vi "Global_All_Data.vi"() -> ()   [LabVIEW 2019]
uses:
  TypeDef/Cluster MISURE.ctl
  TypeDef/MISURE NM.ctl
  TypeDef/Cluster misure ALL.ctl
  TypeDef/Cluster NI.ctl
  cDAQ_PLC Folder/controls/StatoAO_cdaq.ctl
  cDAQ_PLC Folder/controls/statoDO_Cdaq.ctl
  TypeDef/MISURE WT.ctl
  TypeDef/ClusterRes.ctl
  TypeDef/INTERFACCIA.ctl
  TypeDef/Lista AO sistema.ctl
  TypeDef/DOinterfaccia.ctl
  cDAQ_PLC Folder/ST1200_LIST_IO/STATO PLC 1.ctl
  cDAQ_PLC Folder/ST1200_LIST_IO/Uscite PLC 1.ctl
  cDAQ_PLC Folder/controls/statoAO_plc_1.ctl
  cDAQ_PLC Folder/ST1200_LIST_IO/StatoDO_PLC_1.ctl
  SINUS PENTA SANTERNO/controls/Parametri inverter letti.ctl
  cDAQ_PLC Folder/ST1200_LIST_IO/STATO PLC 2.ctl
  cDAQ_PLC Folder/ST1200_LIST_IO/Uscite PLC 2.ctl
  cDAQ_PLC Folder/controls/statoAO_plc_2.ctl
  cDAQ_PLC Folder/ST1200_LIST_IO/StatoDO_PLC_2.ctl
  cDAQ_PLC Folder/ST1200_LIST_IO/STATO PLC 3.ctl
  cDAQ_PLC Folder/ST1200_LIST_IO/Uscite PLC 3.ctl
  cDAQ_PLC Folder/controls/statoAO_plc_3.ctl
  cDAQ_PLC Folder/ST1200_LIST_IO/StatoDO_PLC_3.ctl
  DCREG/Parametri DCREG letti.ctl
panel:
  out "All Data":T1={"MISURE NM"={"Banco"="", "Anno"="", "Numero"="", "Ntabella"="", "Misura"="", "Tipo Prova"="", "ProgressivoAcq"="", "Descrizione"="", "Data_ora"="", "t. acq [h:m:s]"="", "t. acq [min]"="", "t. acq [s]"="", "n [rpm]"="", "f [Hz]"="", "U1[V]"="", "U2 [V]"="", "U3 [V]"="", "U123_media [V]"="", "I1[A]"="", "I2[A]"="", "I3[A]"="", "I123_media [A]*I"="", "I_123_sbil [%]"="", "Ulin[V]"="", "Uc [V]"="", "Uaux [V]"="", "Ilin[A]*I"="", "Imar[A]"="", "Iaux[A]"="", "Uarm[V]"="", "Uecc[V]"="", "Iarm[A]*I"="", "Iecc[A]"="", "pf"="", "P1 [W]"="", "P1 [kW]"="", "Q [VAR]"="", "Q [kVAR]"="", "S [VA]"="", "S [kVA]"="", "P1arm[W]"="", "P1ecc[W]"="", "Parm[kW]"="", "P1ecc[kW]"="", "Cond[uF]"="", "P1_linea_6fili[W]"="", "P1_linea_6fili[kW]"="", "eta_gr_6fili [%]"="", "eta_inverter_6fili [%]"="", "pf_linea_6fili"="", "U4 [V]"="", "U5 [V]"="", "U6 [V]"="", "U456_media [V]"="", "I4 [A]"="", "I5 [A]"="", "I6 [A]"="", "I456_media [A]"="", "C [Nm]*C"="", "Cric [Nm]"="", "Cric\\Cnom"="", "Iric[A]"="", "Iric\\Inom"="", "P2_mecc [W]"="", "P2_mecc [kW]"="", "eta motore [%]"="", "Scorr[%]"="", "Tamb[°C]"="", "R1[ohm]"="", "R2[ohm]"="", "R3[ohm]"="", "Rmedia[ohm]"="", "DT_R1[°C]"="", "DT_R2[°C]"="", "DT_R3[°C]"="", "DT_media[°C]"="", "R_marcia[ohm]"="", "R_aux[ohm]"="", "DT_marcia[°C]"="", "DT_aux[°C]"="", "R_Arm[ohm]"="", "R_Ecc[ohm]"="", "DT_Arm[°C]"="", "DT_Ecc[°C]"="", "TambFreddo[°C]"="", "R1_freddo[ohm]"="", "R2_freddo[ohm]"="", "R3_freddo[ohm]"="", "Rmedia_freddo[ohm]"="", "R_Marcia_freddo[ohm]"="", "R_Aux_freddo[ohm]"="", "R_Arm_freddo[ohm]"="", "R_Ecc_freddo[ohm]"="", "TC1 [°C]"="", "TC2 [°C]"="", "TC3 [°C]"="", "TC4 [°C]"="", "TC5 [°C]"="", "TC6 [°C]"="", "TC7 [°C]"="", "TC8 [°C]"="", "PT1000_1[°C]"="", "PT1000_2[°C]"="", "PT1000_3[°C]"="", "Vdc eccitatrice[V]"="", "Idc eccitatrice[A]"="", "Vdc rotore[V]"="", "Idc rotore[A]"="", "Vac rotore[V]"="", "Iac rotore[V]"="", "V dinamo[V]"="", "Portata Q"="", "Pressione H"="", "U1'[V]"="", "U2'[V]"="", "U3'[V]"="", "I1'[A]"="", "I2'[A]"="", "I3'[A]"="", "U''R-N"="", "U''S-N"="", "U'' T-N"="", "U''R-S"="", "U''R-T"="", "U''S-T"="", "I1''[A]"="", "I2''[A]"="", "I3''[A]"="", "F''[Hz]"="", "P''[kW]"="", "CosFi''"="", "PT1000_4[°C]"="", "Scorta 3"=""}, "MISURE ALL"={"Cluster READ NI"={"AI (0-10V)"={"AI 0"=0.0, "AI 1"=0.0, "AI 2"=0.0, "AI 3"=0.0, "AI 4"=0.0, "AI 5"=0.0, "AI 6"=0.0, "AI 7"=0.0, "AI 8"=0.0, "AI 9"=0.0, "AI 10"=0.0, "AI 11"=0.0, "AI 12"=0.0, "AI 13"=0.0, "AI 14"=0.0, "AI 15"=0.0, "AI 16"=0.0, "AI 17"=0.0, "AI 18"=0.0, "AI 19"=0.0, "AI 20"=0.0, "AI 21"=0.0, "AI 22"=0.0, "AI 23"=0.0, "AI 24"=0.0, "AI 25"=0.0, "AI 26"=0.0, "AI 27"=0.0, "AI 28"=0.0, "AI 29"=0.0, "AI 30"=0.0, "AI 31"=0.0}, "StatoAO_Cdaq[0-10V]"={"AO 1"=0.0, "AO 2"=0.0, "AO 3"=0.0, "AO 4"=0.0}, "Contatori [rpm]"={"RPM 1"=0.0, "RPM 2"=0.0}, "StatoAO_Cdaq [4-20mA]"={"Cdaq_AO [0-10V] 0 for Torque"=0.0, "Cdaq_AO [0-10V] 1"=0.0, "Cdaq_AO [0-10V] 2"=0.0, "Cdaq_AO [0-10V] 3"=0.0}, "StatoDO_Cdaq"={"Scorta 0"=FALSE, "Scorta 1"=FALSE, "Scorta 2"=FALSE, "Scorta 3"=FALSE, "Scorta 4"=FALSE, "Scorta 5"=FALSE, "Scorta 6"=FALSE, "Scorta 7"=FALSE, "Scorta 8"=FALSE, "Scorta 9"=FALSE, "Scorta 10"=FALSE, "Scorta 11"=FALSE, "Scorta 12"=FALSE, "Scorta 13"=FALSE, "Scorta 14"=FALSE, "Scorta 15"=FALSE, "Scorta 16"=FALSE, "Scorta 17"=FALSE, "Scorta 18"=FALSE, "Scorta 19"=FALSE, "Scorta 20"=FALSE, "Scorta 21"=FALSE, "Scorta 22"=FALSE, "Scorta 23"=FALSE, "Scorta 24"=FALSE, "Scorta 25"=FALSE, "Scorta 26"=FALSE, "Scorta 27"=FALSE, "Scorta 28"=FALSE, "Scorta 29"=FALSE, "Scorta 30"=FALSE, "Scorta 31"=FALSE}, "DI"={"Scorta 0"=FALSE, "Scorta 1"=FALSE, "Scorta 2"=FALSE, "Scorta 3"=FALSE, "Scorta 4"=FALSE, "Scorta 5"=FALSE, "Scorta 6"=FALSE, "Scorta 7"=FALSE, "Scorta 8"=FALSE, "Scorta 9"=FALSE, "Scorta 10"=FALSE, "Scorta 11"=FALSE, "Scorta 12"=FALSE, "Scorta 13"=FALSE, "Scorta 14"=FALSE, "Scorta 15"=FALSE, "Scorta 16"=FALSE, "Scorta 17"=FALSE, "Scorta 18"=FALSE, "Scorta 19"=FALSE, "Scorta 20"=FALSE, "Scorta 21"=FALSE, "Scorta 22"=FALSE, "Scorta 23"=FALSE, "Scorta 24"=FALSE, "Scorta 25"=FALSE, "Scorta 26"=FALSE, "Scorta 27"=FALSE, "Scorta 28"=FALSE, "Scorta 29"=FALSE, "Scorta 30"=FALSE, "Scorta 31"=FALSE}, "AI (4-20mA)"={"AI 0"=0.0, "AI 1"=0.0, "AI 2"=0.0, "AI 3"=0.0, "AI 4"=0.0, "AI 5"=0.0, "AI 6"=0.0, "AI 7"=0.0, "AI 8"=0.0, "AI 9"=0.0, "AI 10"=0.0, "AI 11"=0.0, "AI 12"=0.0, "AI 13"=0.0, "AI 14"=0.0, "AI 15"=0.0}, "TC [°C]"={"tc 1"=0.0, "tc 2"=0.0, "tc 3"=0.0, "tc 4"=0.0}, "NI Read Values"={"RPM"=0.0, "Frequency"=0.0, "Mod 1"={"Torsiometro 1"=0.0, "Torsiometro 2"=0.0, "Strin Gauge 1"=0.0, "Strin Gauge 2"=0.0}, "Mod 2"={"Termocoppia 1"=0.0, "Termocoppia 2"=0.0, "Termocoppia 3"=0.0, "Termocoppia 4"=0.0}, "Mod 3"={"PT 100 1"=0.0, "PT 100 2"=0.0, "PT 100 3"=0.0, "PT 100 4"=0.0}}}, "MISURE WT"={"URMS 1"=0.0, "IRMS 1"=0.0, "P 1"=0.0, "S 1"=0.0, "Q 1"=0.0, "LAMBDA 1"=0.0, "PHI 1"=0.0, "F U 1"=0.0, "F I 1"=0.0, "NONE 1"=0.0, "URMS 2"=0.0, "IRMS 2"=0.0, "P 2"=0.0, "S 2"=0.0, "Q 2"=0.0, "LAMBDA 2"=0.0, "PHI 2"=0.0, "F U 2"=0.0, "F I 2"=0.0, "NONE 2"=0.0, "URMS 3"=0.0, "IRMS 3"=0.0, "P 3"=0.0, "S 3"=0.0, "Q 3"=0.0, "LAMBDA 3"=0.0, "PHI 3"=0.0, "F U 3"=0.0, "F I 3"=0.0, "NONE 3"=0.0, "URMS SIGMA"=0.0, "IRMS SIGMA"=0.0, "P SIGMA"=0.0, "S SIGMA"=0.0, "Q SIGMA"=0.0, "LAMBDA SIGMA"=0.0, "PHI SIGMA"=0.0, "F U SIGMA"=0.0, "F I SIGMA"=0.0, "NONE 4"=0.0}, "Resistenze Resistomat"={"Res Ch1"=0.0, "Res Ch2"=0.0, "Res Ch3"=0.0, "Tamb"=0.0}, "INTERFACCIA"={"AI"={"Portate"=[], "Pressioni"=[], "Coppie[Nm]"=[], "Valvole prop %"=[], "RPM"=[], "Livelli"=[], "Temperature"=[], "Riferimenti %"=[], "TENSIONI"=[], "CORRENTI"=[]}, "DI (logici)"={"Start da pulsantiera"=FALSE, "Stop da pulsantiera"=FALSE, "Reset da pulsantiera"=FALSE, "Sistema OK"=FALSE, "Collaudo abilitato"=FALSE, "Potenza trifase abilitata"=FALSE, "Potenza monofase abilitata"=FALSE, "Potenza DC abilitata"=FALSE, "Potenza DC ECC abilitata"=FALSE, "Start alimentazione AC"=FALSE, "Start alimentazione DC"=FALSE, "Start DC eccitazione"=FALSE, "Teleruttore WT abilitato"=FALSE, "Teleruttore Resistomat abilitato"=FALSE, "Teleruttore corto fasi"=FALSE, "Ramo 1 resistomat"=FALSE, "Ramo 2 resistomat"=FALSE, "Ramo 3 resistomat"=FALSE, "B1 Scelta linea elettrica 1"=FALSE, "B1 Scelta linea elettrica 2"=FALSE, "B1 Scelta linea elettrica 3"=FALSE, "B1 Scelta linea elettrica 4"=FALSE, "B1 Scelta linea elettrica 5"=FALSE, "B2 Scelta linea elettrica 1"=FALSE, "B2 Scelta linea elettrica 2"=FALSE, "B2 Scelta linea elettrica 3"=FALSE, "B2 Scelta linea elettrica 4"=FALSE, "B2 Scelta linea elettrica 5"=FALSE, "Rotore bloccato 1"=FALSE, "Rotore bloccato 2"=FALSE, "FRENO 1 abilitato"=FALSE, "FRENO 1 run"=FALSE, "FRENO 1 senso rotaz"=FALSE, "FRENO 1 ctrl velocità"=FALSE, "FRENO 2 abilitato"=FALSE, "FRENO 2 run"=FALSE, "FRENO 2 senso rotaz"=FALSE, "FRENO 2 ctrl velocità"=FALSE, "ALIM 1 abilitato"=FALSE, "ALIM 1 run"=FALSE, "ALIM 2 abilitato"=FALSE, "ALIM 2 run"=FALSE, "ALIM 3 abilitato"=FALSE, "ALIM 3 run"=FALSE, "FRENO 1 ctrl coppia"=FALSE, "FRENO 2 ctrl coppia"=FALSE, "FRENO 3 ctrl coppia"=FALSE, "DI (logici) aggiuntivi impianto"={"Solo freno abilitato"=FALSE, "Carico resistivo abilitato"=FALSE, "AFE+freno abilitato"=FALSE, "Protezioni chiuse"=FALSE, "Start potenza AFE"=FALSE, "AFE in marcia"=FALSE}, "Misura corrente diretta WT"=FALSE, "Misura corrente sens ext"=FALSE, "Sens ext abilitati"=FALSE}, "AO non scalati"={"FRENO1 rif vel"=0.0, "FRENO1 rif Coppia"=0.0, "FRENO2 rif vel"=0.0, "FRENO2 rif Coppia"=0.0, "ALIM1 rif V"=0.0, "ALIM1 rif F"=0.0, "ALIM2 rif V"=0.0, "ALIM2 rif F"=0.0, "ALIM3 rif V"=0.0, "ALIM3 rif F"=0.0, "Fnom keb"=0.0, "Rpm nom keb"=0.0, "Pnom keb"=0.0, "Inom keb"=0.0, "Vnom keb"=0.0, "Rpm max keb"=0.0, "Tempo rampa keb"=0.0, "Tipo Mot keb"=0.0, "FRENO  rif Coppia "=0.0, "FRENO  rif  Corrente"=0.0}, "AO scalati"={"FRENO1 rif vel"=0.0, "FRENO1 rif Coppia"=0.0, "FRENO2 rif vel"=0.0, "FRENO2 rif Coppia"=0.0, "ALIM1 rif V"=0.0, "ALIM1 rif F"=0.0, "ALIM2 rif V"=0.0, "ALIM2 rif F"=0.0, "ALIM3 rif V"=0.0, "ALIM3 rif F"=0.0, "Fnom keb"=0.0, "Rpm nom keb"=0.0, "Pnom keb"=0.0, "Inom keb"=0.0, "Vnom keb"=0.0, "Rpm max keb"=0.0, "Tempo rampa keb"=0.0, "Tipo Mot keb"=0.0, "FRENO  rif Coppia "=0.0, "FRENO  rif  Corrente"=0.0}, "DO (logici)"={"Scelta banco 1"=FALSE, "Scelta banco 2"=FALSE, "Scelta banco 3"=FALSE, "FRENO 1 abilita"=FALSE, "FRENO 1 start"=FALSE, "FRENO 1 senso rotaz"=FALSE, "FRENO 1 ctrl velocità"=FALSE, "FRENO 2 abilita"=FALSE, "FRENO 2 start"=FALSE, "FRENO 2 senso rotaz"=FALSE, "FRENO 2 ctrl velocità"=FALSE, "ALIM 1 abilita"=FALSE, "ALIM 1 start"=FALSE, "ALIM 2 abilita"=FALSE, "ALIM 2 start"=FALSE, "ALIM 3 abilita"=FALSE, "ALIM 3 start"=FALSE, "Abilita linea trifase"=FALSE, "Abilita linea monofase"=FALSE, "Abilita linea dc"=FALSE, "Abilita linea dc eccit"=FALSE, "B1 Linea elettrica 1"=FALSE, "B1 Linea elettrica 2"=FALSE, "B1 Linea elettrica 3"=FALSE, "B1 Linea elettrica 4"=FALSE, "B1 Linea elettrica 5"=FALSE, "B2 Linea elettrica 1"=FALSE, "B2 Linea elettrica 2"=FALSE, "B2 Linea elettrica 3"=FALSE, "B2 Linea elettrica 4"=FALSE, "B2 Linea elettrica 5"=FALSE, "Start potenza AC"=FALSE, "Stop pontenza AC"=FALSE, "Start potenza DC"=FALSE, "Stop potenza DC"=FALSE, "Start potenza eccitaz"=FALSE, "Stop potenza eccitaz"=FALSE, "Reset allarmi"=FALSE, "watchdog"=FALSE, "Scala torsiometro B1"=FALSE, "Controllo torsiom B1"=FALSE, "Scala torsiometro B2"=FALSE, "Controllo torsiom B2"=FALSE, "Teleruttore WT abilita"=FALSE, "Teleruttore Resistomat abilita"=FALSE, "Teleruttore corto fasi"=FALSE, "Ramo 1 resistomat"=FALSE, "Ramo 2 resistomat"=FALSE, "Ramo 3 resistomat"=FALSE, "Collaudo in corso"=FALSE, "Allarme presente"=FALSE, "Enable Res Meter"=FALSE, "Bypass Res Meter"=FALSE, "2nd canale Res Meter"=FALSE, "Scala 200/2000 res meter"=FALSE, "Taratura res meter"=FALSE, "FRENO 1 ctrl coppia"=FALSE, "FRENO 2 ctrl coppia"=FALSE, "FRENO 3 ctrl coppia"=FALSE, "Aggiuntivi impianto"={"Senso rotazione alim 1"=FALSE, "Senso rotazione alim 2"=FALSE}, "ALIM 1 stop"=FALSE, "ALIM 2 stop"=FALSE, "ALIM 3 stop"=FALSE, "FRENO 1 stop"=FALSE, "FRENO 2 stop"=FALSE, "FRENO 3 stop"=FALSE, "B1 configurazione freno B"=FALSE, "B2 configurazione freno B"=FALSE, "Abilita scrittura KEB"=FALSE, "Bench Selection (0-B1,1-B2)"=FALSE, "Select current mode"=FALSE, "Select torque mode"=FALSE, "Select speed mode"=FALSE, "Start"=FALSE, "Stop"=FALSE, "Block"=FALSE, "Enable Force mode"=FALSE, "Abilita linea 125 A"=FALSE, "Abilita linea 63 A"=FALSE, "Abilita linea 16 A"=FALSE, "Aum Tensione Variac"=FALSE, "Dim Tesnione Variac"=FALSE, "Abilita ellectro stractura"=FALSE, "Risprinito Emergence"=FALSE, "Abilita collaudo"=FALSE, "Disabilita collaudo"=FALSE, "External Alaram"=FALSE, "Enable external program"=FALSE, "Reset"=FALSE, "Abilita Ingresso Variac"=FALSE, "Abilita Ventilatore Variac"=FALSE, "Abilita Uscita Variac "=FALSE}}, "FREDDO resistomat"={"Res Ch1"=0.0, "Res Ch2"=0.0, "tAMB"=0.0, "Res Ch3"=0.0}, "STATO PLC 1"={"USCITE PLC"={"AO (real) 2"={"SCORTA 1"=0.0, "SCORTA 2"=0.0, "SCORTA 3"=0.0, "SCORTA 4"=0.0, "SCORTA 5"=0.0, "SCORTA 6"=0.0, "SCORTA 7"=0.0, "SCORTA 8"=0.0}, "statoAO_PLC out"={"Rif Lim coppia freno [%]"=nan, "Rif rpm freno [%]"=nan, "Rif coppia freno [%]"=0.0, "Rif V alimentatore [%]"=0.0, "Rif F alimentatore [%]"=0.0}, "DO (bit)"={"Scelta banco 1"=FALSE, "Set dati motore freno 2"=FALSE, "Diretto inverter"=FALSE, "Filtro LC"=FALSE, "Marcia ALIM (1s)"=FALSE, "Marcia FRENO (1s)"=FALSE, "Stop AFE (1s)"=FALSE, "Stop freno (1s)"=FALSE, "Reset allarmi"=FALSE, "Watchdog"=FALSE, "Senso rotazione"=FALSE, "Abilita collaudo (1s)"=FALSE, "Disabilita collaudo (1s)"=FALSE, "Abilitazione ALIM"=FALSE, "Abilitazione FRENO"=FALSE, "Teleruttore WT"=FALSE, "Senso rot motore prova"=FALSE, "Scorta 7"=FALSE, "Scorta 8"=FALSE, "Scorta 9"=FALSE, "Scorta 10"=FALSE, "Scorta 11"=FALSE, "Scorta 12"=FALSE, "Scorta 13"=FALSE}}, "Stato DI_PLC"={"Sistema OK"=FALSE, "Rotore bloccato"=FALSE, "Scorta 1"=FALSE, "Prova diretto inverter"=FALSE, "Prova con filtro LC"=FALSE, "Teleruttore WT abilitato"=FALSE, "Alim sinus penta abilitato"=FALSE, "Alim sinus penta in marcia"=FALSE, "Freno abilitato"=FALSE, "Freno in marcia"=FALSE, "Senso rotazione freno"=FALSE, "Potenza abilitata"=FALSE, "Scorta 3"=FALSE, "Scorta 4"=FALSE, "scorta 5"=FALSE, "scorta 6"=FALSE}, "AI plc"={"Allarmi 1"=0.0, "Allarmi 2"=0.0, "Scorta 1"=0.0, "Scorta 2"=0.0, "RPM mot prova"=0.0, "I mot prova"=0.0, "RPM freno"=0.0, "I freno"=0.0, "Scorta 3"=0.0, "Scorta 4"=0.0}}, "Res Ch2"=0.0, "Res Ch2 2"=0.0, "FREDDO res meter"={"Res Ch1"=0.0, "Res Ch2"=0.0, "tAMB"=0.0, "Res Ch3"=0.0}, "Resistenze Res Meter"={"Res Ch1"=0.0, "Res Ch2"=0.0, "Res Ch3"=0.0, "Tamb"=0.0}, "READ SINUS PENTA"={"Menù Misure motore (M000-M030)"={"Rif vel a regime (int)"=0, "Rif vel a regime (dec)"=0, "Rif vel dopo rampe (int)"=0, "Rif vel dopo rampe (dec)"=0, "RPM motore (int)"=0, "RPM motore (dec)"=0, "FREQout inverter"=0, "Rif coppia a regime(Nm)"=0, "Richiesta di coppia (Nm)"=0, "Coppia generata dal motore(Nm)"=0, "Rif coppia a regime(%)"=0, "Richiesta di coppia (%)"=0, "Coppia generata dal motore(%)"=0, "Coppia max richiesta prima delle rampe(Nm)"=0, "Coppia max richiesta dopo le rampe(Nm)"=0, "Limite di velocità prima delle rampe"=0, "Limite di velocità dopo le rampe"=0, "Coppia max richiesta prima delle rampe(%)"=0, "Coppia max richiesta dopo le rampe(%)"=0, "Rif di flusso"=0, "Corrente di uscita"=0, "Capacità termica del motore"=0, "Tensione di uscita"=0, "Potenza di uscita"=0, "Energia consumata (LSword)"=0, "Energia consumata (MSword)"=0, "Tensione bus DC"=0, "Tensione di rete"=0}, "Menù regolatore PID (M018-M024)"={"Rif PID a regime(%)"=0, "Rif pid dopo rampe(%)"=0, "Retroazione del pid(%)"=0, "Errore del pid(%)"=0, "uscita del pid(%)"=0, "Rif del pid dopo le rampe"=0, "Retroazione del pid"=0}, "Menù ingressi digitali (M031-M036)"={"Ingressi digitali ritardati"=0, "Ingressi digitali istantanei"=0, "Moresettiera comando loc"=0, "Morsett comando da seriale"=0, "Morsett comando bus di campo"=0, "Ing dig ausiliari da morsettiera"=0, "Ing dig ausiliari da seriale"=0}, "Menù riferimenti (M037-M051)"={"Rif analog est REF"=0, "Rif analog est AIN1"=0, "Rif analog est AIN2"=0, "Rif analog est XAIN4"=0, "Rif analog est XAIN5"=0, "Rif velocità da seriale(int)"=0, "Rif velocità bus di campo(int)"=0, "Rif coppia da seriale"=0, "Rif coppia bus di campo"=0, "Rif del PID da seriale"=0, "Rif del PID da bus di campo"=0, "Retroazione del PID da seriale"=0, "Retroazione del PIDda bus di campo"=0, "Rif da encoder"=0, "Rif in frequenza"=0, "Rif velocità da seriale(dec)"=0, "Rif velocità bus di campo(dec)"=0}, "Menù rampe (P009-P033)"={"Tempo di dec rampa di vel 1"=0, "Tempo di acc rampa di vel 2"=0, "Tempo di dec rampa di vel 2"=0, "Tempo di acc rampa di vel 1"=0, "Unità di mis tempi rampe vel 1/2"=0, "Tempo di acc rampa di vel 3"=0, "Tempo di dec rampa di vel 3"=0, "Tempo di acc rampa di vel 4"=0, "Tempo di dec rampa di vel 4"=0, "Unità di mis tempi rampe vel 3/4"=0, "Selettore arrottondam rampe"=0, "Tempo di arrotond iniz rampa acc"=0, "Tempo di arrotond finale rampa acc"=0, "Tempo di arrotond iniz rampa dec"=0, "Tempo di rampa di salita rif coppia"=0, "Tempo di rampa di discesa rif coppia"=0, "Unità di misura rampa coppia"=0, "Tempo rampa acc marcia jog"=0, "Tempo rampa dec marcia jog"=0, "Reset acc ai cambi pendenza"=0, "rampa di acc in fire mode"=0, "rampa di dec in fire mode"=0, "Tempo di arrotond finale rampa dec"=0}, "Menù controllo motore(C008-C128)"={"Numero motori configurati"=0, "Tipo algoritmo di controllo Mot1"=0, "Tipo rif Mot1"=0, "Tensione nominale rete"=0, "Retroaz di vel da encoder Mot1"=0, "Tipo curva V/f Mot1"=0, "Rotazione delle fasi Mot1"=0, "Freq nominale del motore Mot1"=0, "RPM nominali del motore Mot1"=0, "Potenza nominale del motore Mot1"=0, "Corrente nominale del motore Mot1"=0, "Tensione nominale del motore mot1"=0, "Potenza a vuoto del motore Mot1"=0, "Corrente a vuoto del motore Mot1"=0, "Resistenza statorica del motore Mot1"=0, "Induttanza di dispersione Mot1"=0, "Induttanza mutua motore"=0, "Costante di tempo rotorica"=0, "Costante di tempo filtro pb"=0, "Velocità minima motore"=0, "Velocità massima motore"=0}, "Menù configurazione PID"={"Selezione riferimento n.1"=0, "Selezione retroazione n.1"=0, "Modalità di fuzionamento PID"=0, "Termine derivativo calcolato su err o mis"=0, "Proporz moltiplica deriv e integrale"=0, "Azione del PID"=0}, "ID"=0.0, "Menù uscite digitali"={"MDO4 Inverter pronto"=0}, "Fcarrier"={"Fcarrier Min (Hz)"=0, "Fcarrier Max (Hz)"=0}, "stato inverter M089"=0.0, "Riferimenti"={"Rif tensione"=0, "Rif velocità"=0}, "Comunicazione"=FALSE, "Modalità stop"=0.0}, "STATO PLC 2"={"USCITE PLC"={"AO (real) 2"={"SCORTA 1"=0.0, "SCORTA 2"=0.0, "SCORTA 3"=0.0, "SCORTA 4"=0.0, "SCORTA 5"=0.0, "SCORTA 6"=0.0, "SCORTA 7"=0.0, "SCORTA 8"=0.0}, "statoAO_PLC out"={"Condensatori"=0.0, "Scorta 1"=0.0, "Scorta 2"=0.0}, "DO (bit)"={"Relè misura resistomat"=FALSE, "Misura res ramo 1"=FALSE, "Misura res ramo 2"=FALSE, "Misura res ramo 3"=FALSE, "Scelta banco 2"=FALSE, "Scala Torsiometro"=FALSE, "Ctrl torsiometro"=FALSE, "Select current mode"=FALSE, "Select Torque mode"=FALSE, "Select speed mode"=FALSE, "Watchdog"=FALSE, "Scorta"=FALSE, "Scorta 2"=FALSE, "Scorta 3"=FALSE, "Scorta 4"=FALSE, "Scorta 5"=FALSE, "Bench selection"=FALSE, "External alarm"=FALSE, "Enable external program"=FALSE, "Reset allarmi"=FALSE, "Start"=FALSE, "Stop"=FALSE, "Block"=FALSE, "Scorta 6"=FALSE}}, "Stato DI_PLC"={"Sistema ok"=FALSE, "Relè Resistomat abilitato"=FALSE, "Freno abilitato"=FALSE, "Freno in marcia"=FALSE, "scorta b"=FALSE, "scorta a"=FALSE, "scorta 1"=FALSE, "scorta 2"=FALSE, "scorta 3"=FALSE, "scorta 4"=FALSE, "Scorta 5"=FALSE, "Scorta 6"=FALSE, "Scorta 7"=FALSE, "Scorta 8"=FALSE, "Scorta 9"=FALSE, "Scorta 10"=FALSE}, "AI plc"={"Allarmi 1"=0.0, "Allarmi 2"=0.0, "TC 1"=0.0, "TC 2"=0.0, "TC 3"=0.0, "TC 4"=0.0, "TC 5"=0.0, "TC 6"=0.0, "TC 7"=0.0, "TC 8"=0.0, "PT1000 1"=0.0, "PT1000 2"=0.0, "PT1000 3"=0.0, "PT1000 4"=0.0}}, "STATO PLC 3"={"USCITE PLC"={"AO (real) 2"={"SCORTA 1"=0.0, "SCORTA 2"=0.0, "SCORTA 3"=0.0, "SCORTA 4"=0.0, "SCORTA 5"=0.0, "SCORTA 6"=0.0, "SCORTA 7"=0.0, "SCORTA 8"=0.0}, "statoAO_PLC out"={"Rif velocità alimentatore"=0.0, "Scorta"=0.0, "Tipo Motore  keb"=0.0, "I nom keb"=0.0, "RPM nom keb"=0.0, "V nom keb"=0.0, "F nom keb"=0.0, "t rampa keb"=0.0}, "DO (bit)"={"Select linea Inverter"=FALSE, "Abilita sense wattmetro"=FALSE, "Bypass filtro LC"=FALSE, "Filtro LC"=FALSE, "Bypass trasformatore"=FALSE, "Trasformatore"=FALSE, "Abilita uscite variac"=FALSE, "Abilita linea 125 A"=FALSE, "Abilita linea 63 A"=FALSE, "Abilita linea 16 A"=FALSE, "Abilita Scrittura Dati Keb"=FALSE, "Abilita alimentatore"=FALSE, "Marcia alimentatore (1s)"=FALSE, "Stop alimentatore (1s)"=FALSE, "Senso rot mot prova"=FALSE, "Watchdog"=FALSE, "Aumenta tensione variac"=FALSE, "Diminuisci tensione variac "=FALSE, "Blocco elettroserrature"=FALSE, "Ripristino emergence"=FALSE, "Abilita ingresso variac"=FALSE, "Abilita ventilatore variac"=FALSE, "Reset Allarm"=FALSE, "Scorta 1"=FALSE, "Scorta 2"=FALSE, "Scorta 3"=FALSE, "Scorta 4"=FALSE, "Scorta 5"=FALSE, "Scorta 6"=FALSE, "Scorta 7"=FALSE, "Scorta 8"=FALSE, "Scorta 9"=FALSE, "Abilita collaudo"=FALSE, "Disabilita collaudo "=FALSE, "Scorta 10"=FALSE, "Scorta 11"=FALSE, "Scorta 12"=FALSE, "Scorta 13"=FALSE, "Scorta 14"=FALSE, "Scorta 15"=FALSE}}, "Stato DI_PLC"={"Sistema OK"=FALSE, "Rotore bloccato"=FALSE, "Filtro LC"=FALSE, "Bypass Filtro LC"=FALSE, "Scelta Trasformatore"=FALSE, "Scelta Bypass trasformatore"=FALSE, "Teleruttore wt abilitato"=FALSE, "Alimentatore abilitato"=FALSE, "Alimentatore in marcia"=FALSE, "Scorta 1"=FALSE, "Scorta 2"=FALSE, "Scorta 3"=FALSE, "Potenza abilitata"=FALSE, "Alimentatore in allarme"=FALSE, "Scorta 4"=FALSE, "Conferma dati KEB"=FALSE, "Scorta 5"=FALSE, "Warning Inverter Alimentatore"=FALSE, "Variac Abilitato"=FALSE, "Linea 125 A abilitata"=FALSE, "Linea 63 A abilitata"=FALSE, "Linea 16 A abilitata"=FALSE, "Scorta 6"=FALSE, "Enable force mode"=FALSE}, "AI plc"={"Allarmi 1"=0.0, "Allarmi 2"=0.0, "RPM motore prova"=0.0, "Corrente motore prova"=0.0, "RPM freno"=0.0, "Corrente freno"=0.0, "Tipo motore keb"=0.0, "I nom keb"=0.0, "RPM nom keb"=0.0, "V nom keb"=0.0, "F nom keb"=0.0, "T rampa keb"=0.0, "scorta"=0.0, "Scorta 2"=0.0}}, "DCREG"={"Parametri di misura"={"M000"=0.0, "M001"=0.0, "M002"=0.0, "M003"=0.0, "M004"=0.0, "M005"=0.0, "M006"=0.0, "M007"=0.0, "M008"=0.0, "M009"=0.0, "M010"=0.0, "M011"=0.0, "M012"=0.0, "M013"=0.0, "M014"=0.0, "M015"=0.0, "M016"=0.0, "M017"=0.0, "M018"=0.0, "M019"=0.0, "M020"=0.0, "M021"=0.0, "M022"=0.0, "M023"=0.0, "M024"=0.0, "M025"=0.0, "M026"=0.0, "M027"=0.0, "M028"=0.0, "M029"=0.0, "M030"=0.0, "M031"=0.0}, "Parametri di programmazione"={"P000"=0.0, "P001"=0.0, "P002"=0.0, "P003"=0.0, "P004"=0.0, "P005"=0.0, "P006"=0.0, "P010"=0.0, "P011"=0.0, "P012"=0.0, "P013"=0.0, "P014"=0.0, "P015"=0.0, "P016"=0.0, "P030"=0.0, "P031"=0.0, "P032"=0.0, "P033"=0.0, "P034"=0.0, "P035"=0.0, "P036"=0.0, "P037"=0.0, "P038"=0.0, "P039"=0.0, "P040"=0.0, "P050"=0.0, "P051"=0.0, "P052"=0.0, "P053"=0.0, "P054"=0.0, "P055"=0.0, "P056"=0.0, "P057"=0.0, "P058"=0.0, "P059"=0.0, "P060"=0.0, "P061"=0.0, "P062"=0.0, "P070"=0.0, "P071"=0.0, "P073"=0.0, "P074"=0.0, "P076"=0.0, "P077"=0.0, "P079"=0.0, "P080"=0.0, "P082"=0.0, "P083"=0.0, "P084"=0.0, "P085"=0.0, "P086"=0.0, "P087"=0.0, "P088"=0.0, "P100"=0.0, "P101"=0.0, "P102"=0.0, "P103"=0.0, "P104"=0.0, "P110"=0.0, "P111"=0.0, "P120"=0.0, "P121"=0.0, "P122"=0.0, "P123"=0.0, "P124"=0.0, "P125"=0.0, "P126"=0.0, "P127"=0.0, "P128"=0.0, "P129"=0.0, "P130"=0.0, "P131"=0.0, "P132"=0.0, "P133"=0.0, "P134"=0.0, "P150"=0.0, "P151"=0.0, "P152"=0.0, "P153"=0.0, "P154"=0.0, "P155"=0.0, "P156"=0.0, "P157"=0.0, "P158"=0.0, "P170"=0.0, "P171"=0.0, "P172"=0.0, "P173"=0.0, "P174"=0.0, "P175"=0.0, "P176"=0.0, "P177"=0.0, "P178"=0.0, "P179"=0.0, "P180"=0.0, "P181"=0.0, "P182"=0.0, "P183"=0.0, "P184"=0.0, "P185"=0.0, "P186"=0.0, "P187"=0.0, "P188"=0.0, "P189"=0.0, "P190"=0.0, "P191"=0.0, "P192"=0.0, "P193"=0.0, "P194"=0.0, "P195"=0.0, "P196"=0.0, "P197"=0.0, "P198"=0.0, "P199"=0.0, "P211"=0.0, "P212"=0.0, "P213"=0.0, "P214"=0.0, "P215"=0.0, "P216"=0.0, "P217"=0.0, "P221"=0.0, "P222"=0.0, "P223"=0.0, "P224"=0.0, "P230"=0.0, "P231"=0.0, "P240"=0.0, "P250"=0.0, "P251"=0.0}, "Parametri di configurazione"={"C000"=0.0, "C001"=0.0, "C002"=0.0, "C010"=0.0, "C011"=0.0, "C012"=0.0, "C014"=0.0, "C015"=0.0, "C016"=0.0, "C017"=0.0, "C018"=0.0, "C030"=0.0, "C050"=0.0, "C051"=0.0, "C052"=0.0, "C060"=0.0, "C061"=0.0, "C062"=0.0, "C063"=0.0, "C070"=0.0, "C072"=0.0, "C074"=0.0, "C090"=0.0, "C091"=0.0, "C092"=0.0, "C093"=0.0, "C094"=0.0, "C100"=0.0, "C101"=0.0, "C102"=0.0, "C103"=0.0, "C105"=0.0, "C106"=0.0, "C107"=0.0, "C108"=0.0, "C110"=0.0, "C111"=0.0, "C112"=0.0, "C120"=0.0, "C121"=0.0, "C122"=0.0, "C130"=0.0, "C131"=0.0, "C132"=0.0, "C133"=0.0, "C134"=0.0, "C135"=0.0, "C141"=0.0, "C142"=0.0, "C143"=0.0, "C150"=0.0, "C151"=0.0, "C153"=0.0, "C154"=0.0, "C155"=0.0, "C156"=0.0, "C157"=0.0, "C158"=0.0, "C159"=0.0, "C160"=0.0, "C161"=0.0, "C162"=0.0, "C163"=0.0, "C164"=0.0, "C165"=0.0, "C170"=0.0}, "Codice allarme"=0.0, "Comunicazione"=FALSE}}} {"MISURE ALL"."Cluster READ NI"."AI (4-20mA)"."AI 15" format="%#_6f"; "MISURE ALL"."Cluster READ NI"."AI (4-20mA)"."AI 14" format="%#_6f"; "MISURE ALL"."Cluster READ NI"."AI (4-20mA)"."AI 13" format="%#_6f"; "MISURE ALL"."Cluster READ NI"."AI (4-20mA)"."AI 11" format="%#_6f"; "MISURE ALL"."Cluster READ NI"."AI (4-20mA)"."AI 10" format="%#_6f"; "MISURE ALL"."Cluster READ NI"."AI (4-20mA)"."AI 9" format="%#_6f"; "MISURE ALL"."Cluster READ NI"."AI (4-20mA)"."AI 4" format="%#_6f"; "MISURE ALL"."Cluster READ NI"."AI (4-20mA)"."AI 12" format="%#_6f"; "MISURE ALL"."Cluster READ NI"."AI (4-20mA)"."AI 0" format="%#_6f"; "MISURE ALL"."Cluster READ NI"."AI (4-20mA)"."AI 1" format="%#_6f"; "MISURE ALL"."Cluster READ NI"."AI (4-20mA)"."AI 2" format="%#_6f"; "MISURE ALL"."Cluster READ NI"."AI (4-20mA)"."AI 3" format="%#_6f"; "MISURE ALL"."Cluster READ NI"."AI (4-20mA)"."AI 5" format="%#_6f"; "MISURE ALL"."Cluster READ NI"."AI (4-20mA)"."AI 6" format="%#_6f"; "MISURE ALL"."Cluster READ NI"."AI (4-20mA)"."AI 7" format="%#_6f"; "MISURE ALL"."Cluster READ NI"."AI (4-20mA)"."AI 8" format="%#_6f"; "MISURE ALL"."Cluster READ NI"."AI (0-10V)"."AI 31" format="%#_6f"; "MISURE ALL"."Cluster READ NI"."AI (0-10V)"."AI 30" format="%#_6f"; "MISURE ALL"."Cluster READ NI"."AI (0-10V)"."AI 29" format="%#_6f"; "MISURE ALL"."Cluster READ NI"."AI (0-10V)"."AI 28" format="%#_6f"; "MISURE ALL"."Cluster READ NI"."AI (0-10V)"."AI 27" format="%#_6f"; "MISURE ALL"."Cluster READ NI"."AI (0-10V)"."AI 26" format="%#_6f"; "MISURE ALL"."Cluster READ NI"."AI (0-10V)"."AI 25" format="%#_6f"; "MISURE ALL"."Cluster READ NI"."AI (0-10V)"."AI 24" format="%#_6f"; "MISURE ALL"."Cluster READ NI"."AI (0-10V)"."AI 23" format="%#_6f"; "MISURE ALL"."Cluster READ NI"."AI (0-10V)"."AI 22" format="%#_6f"; "MISURE ALL"."Cluster READ NI"."AI (0-10V)"."AI 21" format="%#_6f"; "MISURE ALL"."Cluster READ NI"."AI (0-10V)"."AI 20" format="%#_6f"; "MISURE ALL"."Cluster READ NI"."AI (0-10V)"."AI 19" format="%#_6f"; "MISURE ALL"."Cluster READ NI"."AI (0-10V)"."AI 18" format="%#_6f"; "MISURE ALL"."Cluster READ NI"."AI (0-10V)"."AI 17" format="%#_6f"; "MISURE ALL"."Cluster READ NI"."AI (0-10V)"."AI 16" format="%#_6f"; "MISURE ALL"."Cluster READ NI"."AI (0-10V)"."AI 15" format="%#_6f"; "MISURE ALL"."Cluster READ NI"."AI (0-10V)"."AI 14" format="%#_6f"; "MISURE ALL"."Cluster READ NI"."AI (0-10V)"."AI 13" format="%#_6f"; "MISURE ALL"."Cluster READ NI"."AI (0-10V)"."AI 11" format="%#_6f"; "MISURE ALL"."Cluster READ NI"."AI (0-10V)"."AI 10" format="%#_6f"; "MISURE ALL"."Cluster READ NI"."AI (0-10V)"."AI 9" format="%#_6f"; "MISURE ALL"."Cluster READ NI"."AI (0-10V)"."AI 4" format="%#_6f"; "MISURE ALL"."Cluster READ NI"."AI (0-10V)"."AI 12" format="%#_6f"; "MISURE ALL"."Cluster READ NI"."AI (0-10V)"."AI 0" format="%#_6f"; "MISURE ALL"."Cluster READ NI"."AI (0-10V)"."AI 1" format="%#_6f"; "MISURE ALL"."Cluster READ NI"."AI (0-10V)"."AI 2" format="%#_6f"; "MISURE ALL"."Cluster READ NI"."AI (0-10V)"."AI 3" format="%#_6f"; "MISURE ALL"."Cluster READ NI"."AI (0-10V)"."AI 5" format="%#_6f"; "MISURE ALL"."Cluster READ NI"."AI (0-10V)"."AI 6" format="%#_6f"; "MISURE ALL"."Cluster READ NI"."AI (0-10V)"."AI 7" format="%#_6f"; "MISURE ALL"."Cluster READ NI"."AI (0-10V)"."AI 8" format="%#_6f"}
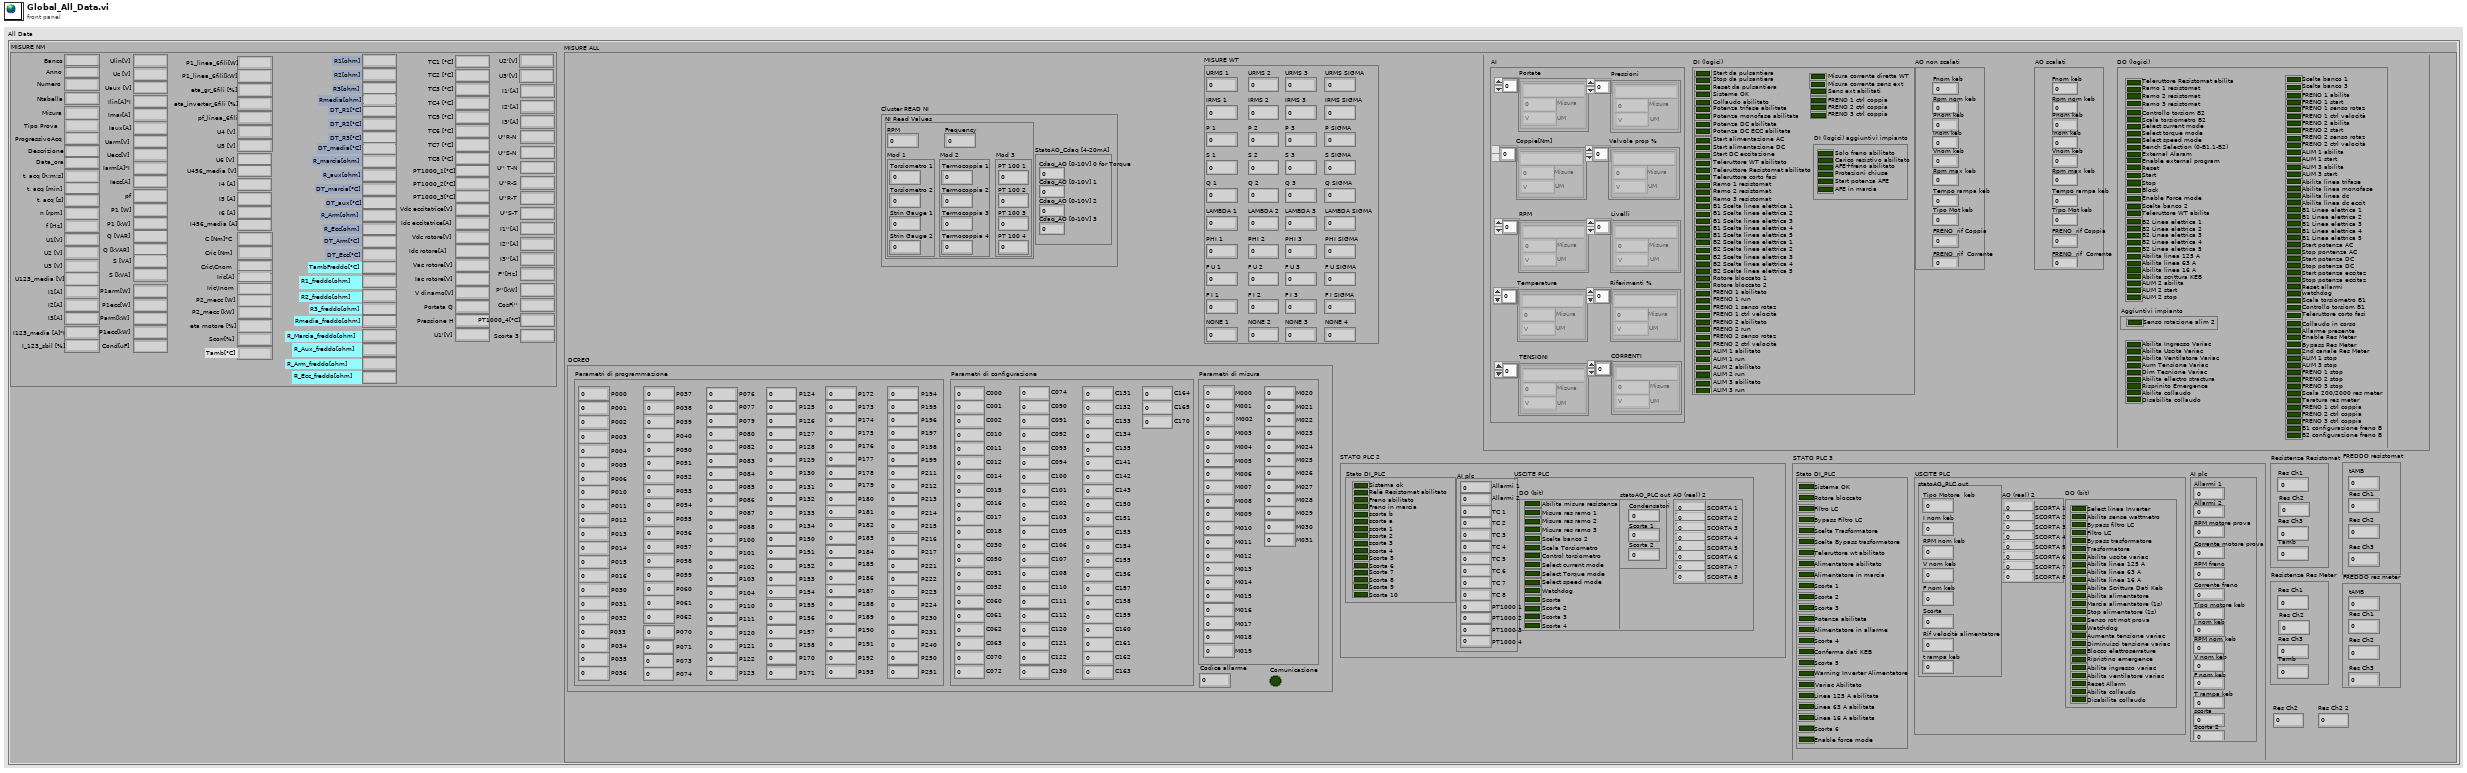
[diagram p1: front panel]
types:
  T1 = typedef "Cluster MISURE.ctl" = cluster{"MISURE NM":T2, "MISURE ALL":T3}
  T2 = typedef "MISURE NM.ctl" = cluster{"Banco":string, "Anno":string, "Numero":string, "Ntabella":string, "Misura":string, "Tipo Prova":string, "ProgressivoAcq":string, "Descrizione":string, "Data_ora":string, "t. acq [h:m:s]":string, "t. acq [min]":string, "t. acq [s]":string, "n [rpm]":string, "f [Hz]":string, "U1[V]":string, "U2 [V]":string, "U3 [V]":string, "U123_media [V]":string, "I1[A]":string, "I2[A]":string, "I3[A]":string, "I123_media [A]*I":string, "I_123_sbil [%]":string, "Ulin[V]":string, "Uc [V]":string, "Uaux [V]":string, "Ilin[A]*I":string, "Imar[A]":string, "Iaux[A]":string, "Uarm[V]":string, "Uecc[V]":string, "Iarm[A]*I":string, "Iecc[A]":string, "pf":string, "P1 [W]":string, "P1 [kW]":string, "Q [VAR]":string, "Q [kVAR]":string, "S [VA]":string, "S [kVA]":string, "P1arm[W]":string, "P1ecc[W]":string, "Parm[kW]":string, "P1ecc[kW]":string, "Cond[uF]":string, "P1_linea_6fili[W]":string, "P1_linea_6fili[kW]":string, "eta_gr_6fili [%]":string, "eta_inverter_6fili [%]":string, "pf_linea_6fili":string, "U4 [V]":string, "U5 [V]":string, "U6 [V]":string, "U456_media [V]":string, "I4 [A]":string, "I5 [A]":string, "I6 [A]":string, "I456_media [A]":string, "C [Nm]*C":string, "Cric [Nm]":string, "Cric\\Cnom":string, "Iric[A]":string, "Iric\\Inom":string, "P2_mecc [W]":string, "P2_mecc [kW]":string, "eta motore [%]":string, "Scorr[%]":string, "Tamb[°C]":string, "R1[ohm]":string, "R2[ohm]":string, "R3[ohm]":string, "Rmedia[ohm]":string, "DT_R1[°C]":string, "DT_R2[°C]":string, "DT_R3[°C]":string, "DT_media[°C]":string, "R_marcia[ohm]":string, "R_aux[ohm]":string, "DT_marcia[°C]":string, "DT_aux[°C]":string, "R_Arm[ohm]":string, "R_Ecc[ohm]":string, "DT_Arm[°C]":string, "DT_Ecc[°C]":string, "TambFreddo[°C]":string, "R1_freddo[ohm]":string, "R2_freddo[ohm]":string, "R3_freddo[ohm]":string, "Rmedia_freddo[ohm]":string, "R_Marcia_freddo[ohm]":string, "R_Aux_freddo[ohm]":string, "R_Arm_freddo[ohm]":string, "R_Ecc_freddo[ohm]":string, "TC1 [°C]":string, "TC2 [°C]":string, "TC3 [°C]":string, "TC4 [°C]":string, "TC5 [°C]":string, "TC6 [°C]":string, "TC7 [°C]":string, "TC8 [°C]":string, "PT1000_1[°C]":string, "PT1000_2[°C]":string, "PT1000_3[°C]":string, "Vdc eccitatrice[V]":string, "Idc eccitatrice[A]":string, "Vdc rotore[V]":string, "Idc rotore[A]":string, "Vac rotore[V]":string, "Iac rotore[V]":string, "V dinamo[V]":string, "Portata Q":string, "Pressione H":string, "U1'[V]":string, "U2'[V]":string, "U3'[V]":string, "I1'[A]":string, "I2'[A]":string, "I3'[A]":string, "U''R-N":string, "U''S-N":string, "U'' T-N":string, "U''R-S":string, "U''R-T":string, "U''S-T":string, "I1''[A]":string, "I2''[A]":string, "I3''[A]":string, "F''[Hz]":string, "P''[kW]":string, "CosFi''":string, "PT1000_4[°C]":string, "Scorta 3":string}
  T3 = typedef "Cluster misure ALL.ctl" = cluster{"Cluster READ NI":T4, "MISURE WT":T7, "Resistenze Resistomat":T8, "INTERFACCIA":T9, "FREDDO resistomat":cluster{"Res Ch1":dbl, "Res Ch2":dbl, "tAMB":dbl, "Res Ch3":dbl}, "STATO PLC 1":T14, "Res Ch2":dbl, "Res Ch2 2":dbl, "FREDDO res meter":cluster{"Res Ch1":dbl, "Res Ch2":dbl, "tAMB":dbl, "Res Ch3":dbl}, "Resistenze Res Meter":T8, "READ SINUS PENTA":T18, "STATO PLC 2":T19, "STATO PLC 3":T23, "DCREG":T27}
  T4 = typedef "Cluster NI.ctl" = cluster{"AI (0-10V)":cluster{"AI 0":dbl, "AI 1":dbl, "AI 2":dbl, "AI 3":dbl, "AI 4":dbl, "AI 5":dbl, "AI 6":dbl, "AI 7":dbl, "AI 8":dbl, "AI 9":dbl, "AI 10":dbl, "AI 11":dbl, "AI 12":dbl, "AI 13":dbl, "AI 14":dbl, "AI 15":dbl, "AI 16":dbl, "AI 17":dbl, "AI 18":dbl, "AI 19":dbl, "AI 20":dbl, "AI 21":dbl, "AI 22":dbl, "AI 23":dbl, "AI 24":dbl, "AI 25":dbl, "AI 26":dbl, "AI 27":dbl, "AI 28":dbl, "AI 29":dbl, "AI 30":dbl, "AI 31":dbl}, "StatoAO_Cdaq[0-10V]":cluster{"AO 1":dbl, "AO 2":dbl, "AO 3":dbl, "AO 4":dbl}, "Contatori [rpm]":cluster{"RPM 1":dbl, "RPM 2":dbl}, "StatoAO_Cdaq [4-20mA]":T5, "StatoDO_Cdaq":T6, "DI":cluster{"Scorta 0":bool, "Scorta 1":bool, "Scorta 2":bool, "Scorta 3":bool, "Scorta 4":bool, "Scorta 5":bool, "Scorta 6":bool, "Scorta 7":bool, "Scorta 8":bool, "Scorta 9":bool, "Scorta 10":bool, "Scorta 11":bool, "Scorta 12":bool, "Scorta 13":bool, "Scorta 14":bool, "Scorta 15":bool, "Scorta 16":bool, "Scorta 17":bool, "Scorta 18":bool, "Scorta 19":bool, "Scorta 20":bool, "Scorta 21":bool, "Scorta 22":bool, "Scorta 23":bool, "Scorta 24":bool, "Scorta 25":bool, "Scorta 26":bool, "Scorta 27":bool, "Scorta 28":bool, "Scorta 29":bool, "Scorta 30":bool, "Scorta 31":bool}, "AI (4-20mA)":cluster{"AI 0":dbl, "AI 1":dbl, "AI 2":dbl, "AI 3":dbl, "AI 4":dbl, "AI 5":dbl, "AI 6":dbl, "AI 7":dbl, "AI 8":dbl, "AI 9":dbl, "AI 10":dbl, "AI 11":dbl, "AI 12":dbl, "AI 13":dbl, "AI 14":dbl, "AI 15":dbl}, "TC [°C]":cluster{"tc 1":dbl, "tc 2":dbl, "tc 3":dbl, "tc 4":dbl}, "NI Read Values":cluster{"RPM":dbl, "Frequency":dbl, "Mod 1":cluster{"Torsiometro 1":dbl, "Torsiometro 2":dbl, "Strin Gauge 1":dbl, "Strin Gauge 2":dbl}, "Mod 2":cluster{"Termocoppia 1":dbl, "Termocoppia 2":dbl, "Termocoppia 3":dbl, "Termocoppia 4":dbl}, "Mod 3":cluster{"PT 100 1":dbl, "PT 100 2":dbl, "PT 100 3":dbl, "PT 100 4":dbl}}}
  T5 = typedef "StatoAO_cdaq.ctl" = cluster{"Cdaq_AO [0-10V] 0 for Torque":dbl, "Cdaq_AO [0-10V] 1":dbl, "Cdaq_AO [0-10V] 2":dbl, "Cdaq_AO [0-10V] 3":dbl}
  T6 = typedef "statoDO_Cdaq.ctl" = cluster{"Scorta 0":bool, "Scorta 1":bool, "Scorta 2":bool, "Scorta 3":bool, "Scorta 4":bool, "Scorta 5":bool, "Scorta 6":bool, "Scorta 7":bool, "Scorta 8":bool, "Scorta 9":bool, "Scorta 10":bool, "Scorta 11":bool, "Scorta 12":bool, "Scorta 13":bool, "Scorta 14":bool, "Scorta 15":bool, "Scorta 16":bool, "Scorta 17":bool, "Scorta 18":bool, "Scorta 19":bool, "Scorta 20":bool, "Scorta 21":bool, "Scorta 22":bool, "Scorta 23":bool, "Scorta 24":bool, "Scorta 25":bool, "Scorta 26":bool, "Scorta 27":bool, "Scorta 28":bool, "Scorta 29":bool, "Scorta 30":bool, "Scorta 31":bool}
  T7 = typedef "MISURE WT.ctl" = cluster{"URMS 1":dbl, "IRMS 1":dbl, "P 1":dbl, "S 1":dbl, "Q 1":dbl, "LAMBDA 1":dbl, "PHI 1":dbl, "F U 1":dbl, "F I 1":dbl, "NONE 1":dbl, "URMS 2":dbl, "IRMS 2":dbl, "P 2":dbl, "S 2":dbl, "Q 2":dbl, "LAMBDA 2":dbl, "PHI 2":dbl, "F U 2":dbl, "F I 2":dbl, "NONE 2":dbl, "URMS 3":dbl, "IRMS 3":dbl, "P 3":dbl, "S 3":dbl, "Q 3":dbl, "LAMBDA 3":dbl, "PHI 3":dbl, "F U 3":dbl, "F I 3":dbl, "NONE 3":dbl, "URMS SIGMA":dbl, "IRMS SIGMA":dbl, "P SIGMA":dbl, "S SIGMA":dbl, "Q SIGMA":dbl, "LAMBDA SIGMA":dbl, "PHI SIGMA":dbl, "F U SIGMA":dbl, "F I SIGMA":dbl, "NONE 4":dbl}
  T8 = typedef "ClusterRes.ctl" = cluster{"Res Ch1":dbl, "Res Ch2":dbl, "Res Ch3":dbl, "Tamb":dbl}
  T9 = typedef "INTERFACCIA.ctl" = cluster{"AI":cluster{"Portate":T10[], "Pressioni":T10[], "Coppie[Nm]":T10[], "Valvole prop %":T10[], "RPM":T10[], "Livelli":T10[], "Temperature":T10[], "Riferimenti %":T10[], "TENSIONI":T10[], "CORRENTI":T10[]}, "DI (logici)":cluster{"Start da pulsantiera":bool, "Stop da pulsantiera":bool, "Reset da pulsantiera":bool, "Sistema OK":bool, "Collaudo abilitato":bool, "Potenza trifase abilitata":bool, "Potenza monofase abilitata":bool, "Potenza DC abilitata":bool, "Potenza DC ECC abilitata":bool, "Start alimentazione AC":bool, "Start alimentazione DC":bool, "Start DC eccitazione":bool, "Teleruttore WT abilitato":bool, "Teleruttore Resistomat abilitato":bool, "Teleruttore corto fasi":bool, "Ramo 1 resistomat":bool, "Ramo 2 resistomat":bool, "Ramo 3 resistomat":bool, "B1 Scelta linea elettrica 1":bool, "B1 Scelta linea elettrica 2":bool, "B1 Scelta linea elettrica 3":bool, "B1 Scelta linea elettrica 4":bool, "B1 Scelta linea elettrica 5":bool, "B2 Scelta linea elettrica 1":bool, "B2 Scelta linea elettrica 2":bool, "B2 Scelta linea elettrica 3":bool, "B2 Scelta linea elettrica 4":bool, "B2 Scelta linea elettrica 5":bool, "Rotore bloccato 1":bool, "Rotore bloccato 2":bool, "FRENO 1 abilitato":bool, "FRENO 1 run":bool, "FRENO 1 senso rotaz":bool, "FRENO 1 ctrl velocità":bool, "FRENO 2 abilitato":bool, "FRENO 2 run":bool, "FRENO 2 senso rotaz":bool, "FRENO 2 ctrl velocità":bool, "ALIM 1 abilitato":bool, "ALIM 1 run":bool, "ALIM 2 abilitato":bool, "ALIM 2 run":bool, "ALIM 3 abilitato":bool, "ALIM 3 run":bool, "FRENO 1 ctrl coppia":bool, "FRENO 2 ctrl coppia":bool, "FRENO 3 ctrl coppia":bool, "DI (logici) aggiuntivi impianto":cluster{"Solo freno abilitato":bool, "Carico resistivo abilitato":bool, "AFE+freno abilitato":bool, "Protezioni chiuse":bool, "Start potenza AFE":bool, "AFE in marcia":bool}, "Misura corrente diretta WT":bool, "Misura corrente sens ext":bool, "Sens ext abilitati":bool}, "AO non scalati":T12, "AO scalati":T12, "DO (logici)":T13}
  T10 = typedef "ClusterMisura_e_Unità_INPUT.ctl" = cluster{"Misura":dbl, "UM":T11, "Descrizione":string}
  T11 = typedef "UnitàMisura.ctl" = enum16{"V", "mA", "Bar", "RPM", "m3/s", "m3/min", "m3/h", "l/s", "l/min", "in3/min", "ft3/min", "gpm", "igpm", "igph", "%", "°C", "m", "Nm", "A"}
  T12 = typedef "Lista AO sistema.ctl" = cluster{"FRENO1 rif vel":dbl, "FRENO1 rif Coppia":dbl, "FRENO2 rif vel":dbl, "FRENO2 rif Coppia":dbl, "ALIM1 rif V":dbl, "ALIM1 rif F":dbl, "ALIM2 rif V":dbl, "ALIM2 rif F":dbl, "ALIM3 rif V":dbl, "ALIM3 rif F":dbl, "Fnom keb":dbl, "Rpm nom keb":dbl, "Pnom keb":dbl, "Inom keb":dbl, "Vnom keb":dbl, "Rpm max keb":dbl, "Tempo rampa keb":dbl, "Tipo Mot keb":dbl, "FRENO  rif Coppia ":dbl, "FRENO  rif  Corrente":dbl}
  T13 = typedef "DOinterfaccia.ctl" = cluster{"Scelta banco 1":bool, "Scelta banco 2":bool, "Scelta banco 3":bool, "FRENO 1 abilita":bool, "FRENO 1 start":bool, "FRENO 1 senso rotaz":bool, "FRENO 1 ctrl velocità":bool, "FRENO 2 abilita":bool, "FRENO 2 start":bool, "FRENO 2 senso rotaz":bool, "FRENO 2 ctrl velocità":bool, "ALIM 1 abilita":bool, "ALIM 1 start":bool, "ALIM 2 abilita":bool, "ALIM 2 start":bool, "ALIM 3 abilita":bool, "ALIM 3 start":bool, "Abilita linea trifase":bool, "Abilita linea monofase":bool, "Abilita linea dc":bool, "Abilita linea dc eccit":bool, "B1 Linea elettrica 1":bool, "B1 Linea elettrica 2":bool, "B1 Linea elettrica 3":bool, "B1 Linea elettrica 4":bool, "B1 Linea elettrica 5":bool, "B2 Linea elettrica 1":bool, "B2 Linea elettrica 2":bool, "B2 Linea elettrica 3":bool, "B2 Linea elettrica 4":bool, "B2 Linea elettrica 5":bool, "Start potenza AC":bool, "Stop pontenza AC":bool, "Start potenza DC":bool, "Stop potenza DC":bool, "Start potenza eccitaz":bool, "Stop potenza eccitaz":bool, "Reset allarmi":bool, "watchdog":bool, "Scala torsiometro B1":bool, "Controllo torsiom B1":bool, "Scala torsiometro B2":bool, "Controllo torsiom B2":bool, "Teleruttore WT abilita":bool, "Teleruttore Resistomat abilita":bool, "Teleruttore corto fasi":bool, "Ramo 1 resistomat":bool, "Ramo 2 resistomat":bool, "Ramo 3 resistomat":bool, "Collaudo in corso":bool, "Allarme presente":bool, "Enable Res Meter":bool, "Bypass Res Meter":bool, "2nd canale Res Meter":bool, "Scala 200/2000 res meter":bool, "Taratura res meter":bool, "FRENO 1 ctrl coppia":bool, "FRENO 2 ctrl coppia":bool, "FRENO 3 ctrl coppia":bool, "Aggiuntivi impianto":cluster{"Senso rotazione alim 1":bool, "Senso rotazione alim 2":bool}, "ALIM 1 stop":bool, "ALIM 2 stop":bool, "ALIM 3 stop":bool, "FRENO 1 stop":bool, "FRENO 2 stop":bool, "FRENO 3 stop":bool, "B1 configurazione freno B":bool, "B2 configurazione freno B":bool, "Abilita scrittura KEB":bool, "Bench Selection (0-B1,1-B2)":bool, "Select current mode":bool, "Select torque mode":bool, "Select speed mode":bool, "Start":bool, "Stop":bool, "Block":bool, "Enable Force mode":bool, "Abilita linea 125 A":bool, "Abilita linea 63 A":bool, "Abilita linea 16 A":bool, "Aum Tensione Variac":bool, "Dim Tesnione Variac":bool, "Abilita ellectro stractura":bool, "Risprinito Emergence":bool, "Abilita collaudo":bool, "Disabilita collaudo":bool, "External Alaram":bool, "Enable external program":bool, "Reset":bool, "Abilita Ingresso Variac":bool, "Abilita Ventilatore Variac":bool, "Abilita Uscita Variac ":bool}
  T14 = typedef "STATO PLC 1.ctl" = cluster{"USCITE PLC":T15, "Stato DI_PLC":cluster{"Sistema OK":bool, "Rotore bloccato":bool, "Scorta 1":bool, "Prova diretto inverter":bool, "Prova con filtro LC":bool, "Teleruttore WT abilitato":bool, "Alim sinus penta abilitato":bool, "Alim sinus penta in marcia":bool, "Freno abilitato":bool, "Freno in marcia":bool, "Senso rotazione freno":bool, "Potenza abilitata":bool, "Scorta 3":bool, "Scorta 4":bool, "scorta 5":bool, "scorta 6":bool}, "AI plc":cluster{"Allarmi 1":dbl, "Allarmi 2":dbl, "Scorta 1":dbl, "Scorta 2":dbl, "RPM mot prova":dbl, "I mot prova":dbl, "RPM freno":dbl, "I freno":dbl, "Scorta 3":dbl, "Scorta 4":dbl}}
  T15 = typedef "Uscite PLC 1.ctl" = cluster{"AO (real) 2":cluster{"SCORTA 1":dbl, "SCORTA 2":dbl, "SCORTA 3":dbl, "SCORTA 4":dbl, "SCORTA 5":dbl, "SCORTA 6":dbl, "SCORTA 7":dbl, "SCORTA 8":dbl}, "statoAO_PLC out":T16, "DO (bit)":T17}
  T16 = typedef "statoAO_plc_1.ctl" = cluster{"Rif Lim coppia freno [%]":dbl, "Rif rpm freno [%]":dbl, "Rif coppia freno [%]":dbl, "Rif V alimentatore [%]":dbl, "Rif F alimentatore [%]":dbl}
  T17 = typedef "StatoDO_PLC_1.ctl" = cluster{"Scelta banco 1":bool, "Set dati motore freno 2":bool, "Diretto inverter":bool, "Filtro LC":bool, "Marcia ALIM (1s)":bool, "Marcia FRENO (1s)":bool, "Stop AFE (1s)":bool, "Stop freno (1s)":bool, "Reset allarmi":bool, "Watchdog":bool, "Senso rotazione":bool, "Abilita collaudo (1s)":bool, "Disabilita collaudo (1s)":bool, "Abilitazione ALIM":bool, "Abilitazione FRENO":bool, "Teleruttore WT":bool, "Senso rot motore prova":bool, "Scorta 7":bool, "Scorta 8":bool, "Scorta 9":bool, "Scorta 10":bool, "Scorta 11":bool, "Scorta 12":bool, "Scorta 13":bool}
  T18 = typedef "Parametri inverter letti.ctl" = cluster{"Menù Misure motore (M000-M030)":cluster{"Rif vel a regime (int)":u16, "Rif vel a regime (dec)":u16, "Rif vel dopo rampe (int)":u16, "Rif vel dopo rampe (dec)":u16, "RPM motore (int)":u16, "RPM motore (dec)":u16, "FREQout inverter":u16, "Rif coppia a regime(Nm)":u16, "Richiesta di coppia (Nm)":u16, "Coppia generata dal motore(Nm)":u16, "Rif coppia a regime(%)":u16, "Richiesta di coppia (%)":u16, "Coppia generata dal motore(%)":u16, "Coppia max richiesta prima delle rampe(Nm)":u16, "Coppia max richiesta dopo le rampe(Nm)":u16, "Limite di velocità prima delle rampe":u16, "Limite di velocità dopo le rampe":u16, "Coppia max richiesta prima delle rampe(%)":u16, "Coppia max richiesta dopo le rampe(%)":u16, "Rif di flusso":u16, "Corrente di uscita":u16, "Capacità termica del motore":u16, "Tensione di uscita":u16, "Potenza di uscita":u16, "Energia consumata (LSword)":u16, "Energia consumata (MSword)":u16, "Tensione bus DC":u16, "Tensione di rete":u16}, "Menù regolatore PID (M018-M024)":cluster{"Rif PID a regime(%)":u16, "Rif pid dopo rampe(%)":u16, "Retroazione del pid(%)":u16, "Errore del pid(%)":u16, "uscita del pid(%)":u16, "Rif del pid dopo le rampe":u16, "Retroazione del pid":u16}, "Menù ingressi digitali (M031-M036)":cluster{"Ingressi digitali ritardati":u16, "Ingressi digitali istantanei":u16, "Moresettiera comando loc":u16, "Morsett comando da seriale":u16, "Morsett comando bus di campo":u16, "Ing dig ausiliari da morsettiera":u16, "Ing dig ausiliari da seriale":u16}, "Menù riferimenti (M037-M051)":cluster{"Rif analog est REF":u16, "Rif analog est AIN1":u16, "Rif analog est AIN2":u16, "Rif analog est XAIN4":u16, "Rif analog est XAIN5":u16, "Rif velocità da seriale(int)":u16, "Rif velocità bus di campo(int)":u16, "Rif coppia da seriale":u16, "Rif coppia bus di campo":u16, "Rif del PID da seriale":u16, "Rif del PID da bus di campo":u16, "Retroazione del PID da seriale":u16, "Retroazione del PIDda bus di campo":u16, "Rif da encoder":u16, "Rif in frequenza":u16, "Rif velocità da seriale(dec)":u16, "Rif velocità bus di campo(dec)":u16}, "Menù rampe (P009-P033)":cluster{"Tempo di dec rampa di vel 1":u16, "Tempo di acc rampa di vel 2":u16, "Tempo di dec rampa di vel 2":u16, "Tempo di acc rampa di vel 1":u16, "Unità di mis tempi rampe vel 1/2":u16, "Tempo di acc rampa di vel 3":u16, "Tempo di dec rampa di vel 3":u16, "Tempo di acc rampa di vel 4":u16, "Tempo di dec rampa di vel 4":u16, "Unità di mis tempi rampe vel 3/4":u16, "Selettore arrottondam rampe":u16, "Tempo di arrotond iniz rampa acc":u16, "Tempo di arrotond finale rampa acc":u16, "Tempo di arrotond iniz rampa dec":u16, "Tempo di rampa di salita rif coppia":u16, "Tempo di rampa di discesa rif coppia":u16, "Unità di misura rampa coppia":u16, "Tempo rampa acc marcia jog":u16, "Tempo rampa dec marcia jog":u16, "Reset acc ai cambi pendenza":u16, "rampa di acc in fire mode":u16, "rampa di dec in fire mode":u16, "Tempo di arrotond finale rampa dec":u16}, "Menù controllo motore(C008-C128)":cluster{"Numero motori configurati":u16, "Tipo algoritmo di controllo Mot1":u16, "Tipo rif Mot1":u16, "Tensione nominale rete":u16, "Retroaz di vel da encoder Mot1":u16, "Tipo curva V/f Mot1":u16, "Rotazione delle fasi Mot1":u16, "Freq nominale del motore Mot1":u16, "RPM nominali del motore Mot1":u16, "Potenza nominale del motore Mot1":u16, "Corrente nominale del motore Mot1":u16, "Tensione nominale del motore mot1":u16, "Potenza a vuoto del motore Mot1":u16, "Corrente a vuoto del motore Mot1":u16, "Resistenza statorica del motore Mot1":u16, "Induttanza di dispersione Mot1":u16, "Induttanza mutua motore":u16, "Costante di tempo rotorica":u16, "Costante di tempo filtro pb":u16, "Velocità minima motore":u16, "Velocità massima motore":u16}, "Menù configurazione PID":cluster{"Selezione riferimento n.1":u16, "Selezione retroazione n.1":u16, "Modalità di fuzionamento PID":u16, "Termine derivativo calcolato su err o mis":u16, "Proporz moltiplica deriv e integrale":u16, "Azione del PID":u16}, "ID":dbl, "Menù uscite digitali":cluster{"MDO4 Inverter pronto":u16}, "Fcarrier":cluster{"Fcarrier Min (Hz)":u16, "Fcarrier Max (Hz)":u16}, "stato inverter M089":dbl, "Riferimenti":cluster{"Rif tensione":u16, "Rif velocità":u16}, "Comunicazione":bool, "Modalità stop":dbl}
  T19 = typedef "STATO PLC 2.ctl" = cluster{"USCITE PLC":T20, "Stato DI_PLC":cluster{"Sistema ok":bool, "Relè Resistomat abilitato":bool, "Freno abilitato":bool, "Freno in marcia":bool, "scorta b":bool, "scorta a":bool, "scorta 1":bool, "scorta 2":bool, "scorta 3":bool, "scorta 4":bool, "Scorta 5":bool, "Scorta 6":bool, "Scorta 7":bool, "Scorta 8":bool, "Scorta 9":bool, "Scorta 10":bool}, "AI plc":cluster{"Allarmi 1":dbl, "Allarmi 2":dbl, "TC 1":dbl, "TC 2":dbl, "TC 3":dbl, "TC 4":dbl, "TC 5":dbl, "TC 6":dbl, "TC 7":dbl, "TC 8":dbl, "PT1000 1":dbl, "PT1000 2":dbl, "PT1000 3":dbl, "PT1000 4":dbl}}
  T20 = typedef "Uscite PLC 2.ctl" = cluster{"AO (real) 2":cluster{"SCORTA 1":dbl, "SCORTA 2":dbl, "SCORTA 3":dbl, "SCORTA 4":dbl, "SCORTA 5":dbl, "SCORTA 6":dbl, "SCORTA 7":dbl, "SCORTA 8":dbl}, "statoAO_PLC out":T21, "DO (bit)":T22}
  T21 = typedef "statoAO_plc_2.ctl" = cluster{"Condensatori":dbl, "Scorta 1":dbl, "Scorta 2":dbl}
  T22 = typedef "StatoDO_PLC_2.ctl" = cluster{"Relè misura resistomat":bool, "Misura res ramo 1":bool, "Misura res ramo 2":bool, "Misura res ramo 3":bool, "Scelta banco 2":bool, "Scala Torsiometro":bool, "Ctrl torsiometro":bool, "Select current mode":bool, "Select Torque mode":bool, "Select speed mode":bool, "Watchdog":bool, "Scorta":bool, "Scorta 2":bool, "Scorta 3":bool, "Scorta 4":bool, "Scorta 5":bool, "Bench selection":bool, "External alarm":bool, "Enable external program":bool, "Reset allarmi":bool, "Start":bool, "Stop":bool, "Block":bool, "Scorta 6":bool}
  T23 = typedef "STATO PLC 3.ctl" = cluster{"USCITE PLC":T24, "Stato DI_PLC":cluster{"Sistema OK":bool, "Rotore bloccato":bool, "Filtro LC":bool, "Bypass Filtro LC":bool, "Scelta Trasformatore":bool, "Scelta Bypass trasformatore":bool, "Teleruttore wt abilitato":bool, "Alimentatore abilitato":bool, "Alimentatore in marcia":bool, "Scorta 1":bool, "Scorta 2":bool, "Scorta 3":bool, "Potenza abilitata":bool, "Alimentatore in allarme":bool, "Scorta 4":bool, "Conferma dati KEB":bool, "Scorta 5":bool, "Warning Inverter Alimentatore":bool, "Variac Abilitato":bool, "Linea 125 A abilitata":bool, "Linea 63 A abilitata":bool, "Linea 16 A abilitata":bool, "Scorta 6":bool, "Enable force mode":bool}, "AI plc":cluster{"Allarmi 1":dbl, "Allarmi 2":dbl, "RPM motore prova":dbl, "Corrente motore prova":dbl, "RPM freno":dbl, "Corrente freno":dbl, "Tipo motore keb":dbl, "I nom keb":dbl, "RPM nom keb":dbl, "V nom keb":dbl, "F nom keb":dbl, "T rampa keb":dbl, "scorta":dbl, "Scorta 2":dbl}}
  T24 = typedef "Uscite PLC 3.ctl" = cluster{"AO (real) 2":cluster{"SCORTA 1":dbl, "SCORTA 2":dbl, "SCORTA 3":dbl, "SCORTA 4":dbl, "SCORTA 5":dbl, "SCORTA 6":dbl, "SCORTA 7":dbl, "SCORTA 8":dbl}, "statoAO_PLC out":T25, "DO (bit)":T26}
  T25 = typedef "statoAO_plc_3.ctl" = cluster{"Rif velocità alimentatore":dbl, "Scorta":dbl, "Tipo Motore  keb":dbl, "I nom keb":dbl, "RPM nom keb":dbl, "V nom keb":dbl, "F nom keb":dbl, "t rampa keb":dbl}
  T26 = typedef "StatoDO_PLC_3.ctl" = cluster{"Select linea Inverter":bool, "Abilita sense wattmetro":bool, "Bypass filtro LC":bool, "Filtro LC":bool, "Bypass trasformatore":bool, "Trasformatore":bool, "Abilita uscite variac":bool, "Abilita linea 125 A":bool, "Abilita linea 63 A":bool, "Abilita linea 16 A":bool, "Abilita Scrittura Dati Keb":bool, "Abilita alimentatore":bool, "Marcia alimentatore (1s)":bool, "Stop alimentatore (1s)":bool, "Senso rot mot prova":bool, "Watchdog":bool, "Aumenta tensione variac":bool, "Diminuisci tensione variac ":bool, "Blocco elettroserrature":bool, "Ripristino emergence":bool, "Abilita ingresso variac":bool, "Abilita ventilatore variac":bool, "Reset Allarm":bool, "Scorta 1":bool, "Scorta 2":bool, "Scorta 3":bool, "Scorta 4":bool, "Scorta 5":bool, "Scorta 6":bool, "Scorta 7":bool, "Scorta 8":bool, "Scorta 9":bool, "Abilita collaudo":bool, "Disabilita collaudo ":bool, "Scorta 10":bool, "Scorta 11":bool, "Scorta 12":bool, "Scorta 13":bool, "Scorta 14":bool, "Scorta 15":bool}
  T27 = typedef "Parametri DCREG letti.ctl" = cluster{"Parametri di misura":cluster{"M000":dbl, "M001":dbl, "M002":dbl, "M003":dbl, "M004":dbl, "M005":dbl, "M006":dbl, "M007":dbl, "M008":dbl, "M009":dbl, "M010":dbl, "M011":dbl, "M012":dbl, "M013":dbl, "M014":dbl, "M015":dbl, "M016":dbl, "M017":dbl, "M018":dbl, "M019":dbl, "M020":dbl, "M021":dbl, "M022":dbl, "M023":dbl, "M024":dbl, "M025":dbl, "M026":dbl, "M027":dbl, "M028":dbl, "M029":dbl, "M030":dbl, "M031":dbl}, "Parametri di programmazione":cluster{"P000":dbl, "P001":dbl, "P002":dbl, "P003":dbl, "P004":dbl, "P005":dbl, "P006":dbl, "P010":dbl, "P011":dbl, "P012":dbl, "P013":dbl, "P014":dbl, "P015":dbl, "P016":dbl, "P030":dbl, "P031":dbl, "P032":dbl, "P033":dbl, "P034":dbl, "P035":dbl, "P036":dbl, "P037":dbl, "P038":dbl, "P039":dbl, "P040":dbl, "P050":dbl, "P051":dbl, "P052":dbl, "P053":dbl, "P054":dbl, "P055":dbl, "P056":dbl, "P057":dbl, "P058":dbl, "P059":dbl, "P060":dbl, "P061":dbl, "P062":dbl, "P070":dbl, "P071":dbl, "P073":dbl, "P074":dbl, "P076":dbl, "P077":dbl, "P079":dbl, "P080":dbl, "P082":dbl, "P083":dbl, "P084":dbl, "P085":dbl, "P086":dbl, "P087":dbl, "P088":dbl, "P100":dbl, "P101":dbl, "P102":dbl, "P103":dbl, "P104":dbl, "P110":dbl, "P111":dbl, "P120":dbl, "P121":dbl, "P122":dbl, "P123":dbl, "P124":dbl, "P125":dbl, "P126":dbl, "P127":dbl, "P128":dbl, "P129":dbl, "P130":dbl, "P131":dbl, "P132":dbl, "P133":dbl, "P134":dbl, "P150":dbl, "P151":dbl, "P152":dbl, "P153":dbl, "P154":dbl, "P155":dbl, "P156":dbl, "P157":dbl, "P158":dbl, "P170":dbl, "P171":dbl, "P172":dbl, "P173":dbl, "P174":dbl, "P175":dbl, "P176":dbl, "P177":dbl, "P178":dbl, "P179":dbl, "P180":dbl, "P181":dbl, "P182":dbl, "P183":dbl, "P184":dbl, "P185":dbl, "P186":dbl, "P187":dbl, "P188":dbl, "P189":dbl, "P190":dbl, "P191":dbl, "P192":dbl, "P193":dbl, "P194":dbl, "P195":dbl, "P196":dbl, "P197":dbl, "P198":dbl, "P199":dbl, "P211":dbl, "P212":dbl, "P213":dbl, "P214":dbl, "P215":dbl, "P216":dbl, "P217":dbl, "P221":dbl, "P222":dbl, "P223":dbl, "P224":dbl, "P230":dbl, "P231":dbl, "P240":dbl, "P250":dbl, "P251":dbl}, "Parametri di configurazione":cluster{"C000":dbl, "C001":dbl, "C002":dbl, "C010":dbl, "C011":dbl, "C012":dbl, "C014":dbl, "C015":dbl, "C016":dbl, "C017":dbl, "C018":dbl, "C030":dbl, "C050":dbl, "C051":dbl, "C052":dbl, "C060":dbl, "C061":dbl, "C062":dbl, "C063":dbl, "C070":dbl, "C072":dbl, "C074":dbl, "C090":dbl, "C091":dbl, "C092":dbl, "C093":dbl, "C094":dbl, "C100":dbl, "C101":dbl, "C102":dbl, "C103":dbl, "C105":dbl, "C106":dbl, "C107":dbl, "C108":dbl, "C110":dbl, "C111":dbl, "C112":dbl, "C120":dbl, "C121":dbl, "C122":dbl, "C130":dbl, "C131":dbl, "C132":dbl, "C133":dbl, "C134":dbl, "C135":dbl, "C141":dbl, "C142":dbl, "C143":dbl, "C150":dbl, "C151":dbl, "C153":dbl, "C154":dbl, "C155":dbl, "C156":dbl, "C157":dbl, "C158":dbl, "C159":dbl, "C160":dbl, "C161":dbl, "C162":dbl, "C163":dbl, "C164":dbl, "C165":dbl, "C170":dbl}, "Codice allarme":dbl, "Comunicazione":bool}
diagram:
